vi "AlarmInterFace.vi"() -> ()   [LabVIEW 2015]
uses:
  <userlib>/QMH/Message Queue/Support/Enqueue Message (Single).vi
  <vilib>/Utility/error.llb/Error Cluster From Error Code.vi
  <vilib>/ErrorRing/Error Ring.xnode
  <userlib>/QMH/User Event - Stop/User Event - Stop.lvlib
  <userlib>/QMH/Message Queue/Message Queue.lvlib
panel:
  in  "报警声音消音":bool
  in  "确认所选报警":bool
  in  "确认当前画面所有报警":bool
  in  "AlarmMassge":i32(listbox)
  in  "Exit":bool
  in  "HostThread":variant
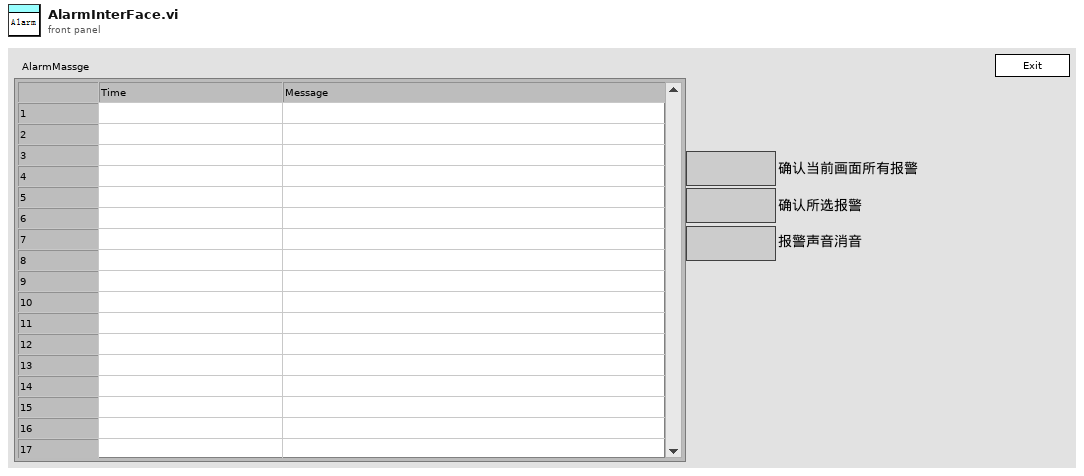
[diagram p1: front panel]
types:
  T1 = cluster{"Controls":cluster{"Exit":refnum<vi>, "AlarmMassge":refnum<vi>}, "Thread":cluster{"ThisQ":string, "ThisVI":refnum<vi>, "HostQ":string, "HostRef":refnum<vi>, "SlavesQ":string[], "SlavesRef":refnum<vi>[]}, "Data":cluster{"Replace":bool}, "User":cluster{"Name":string}}
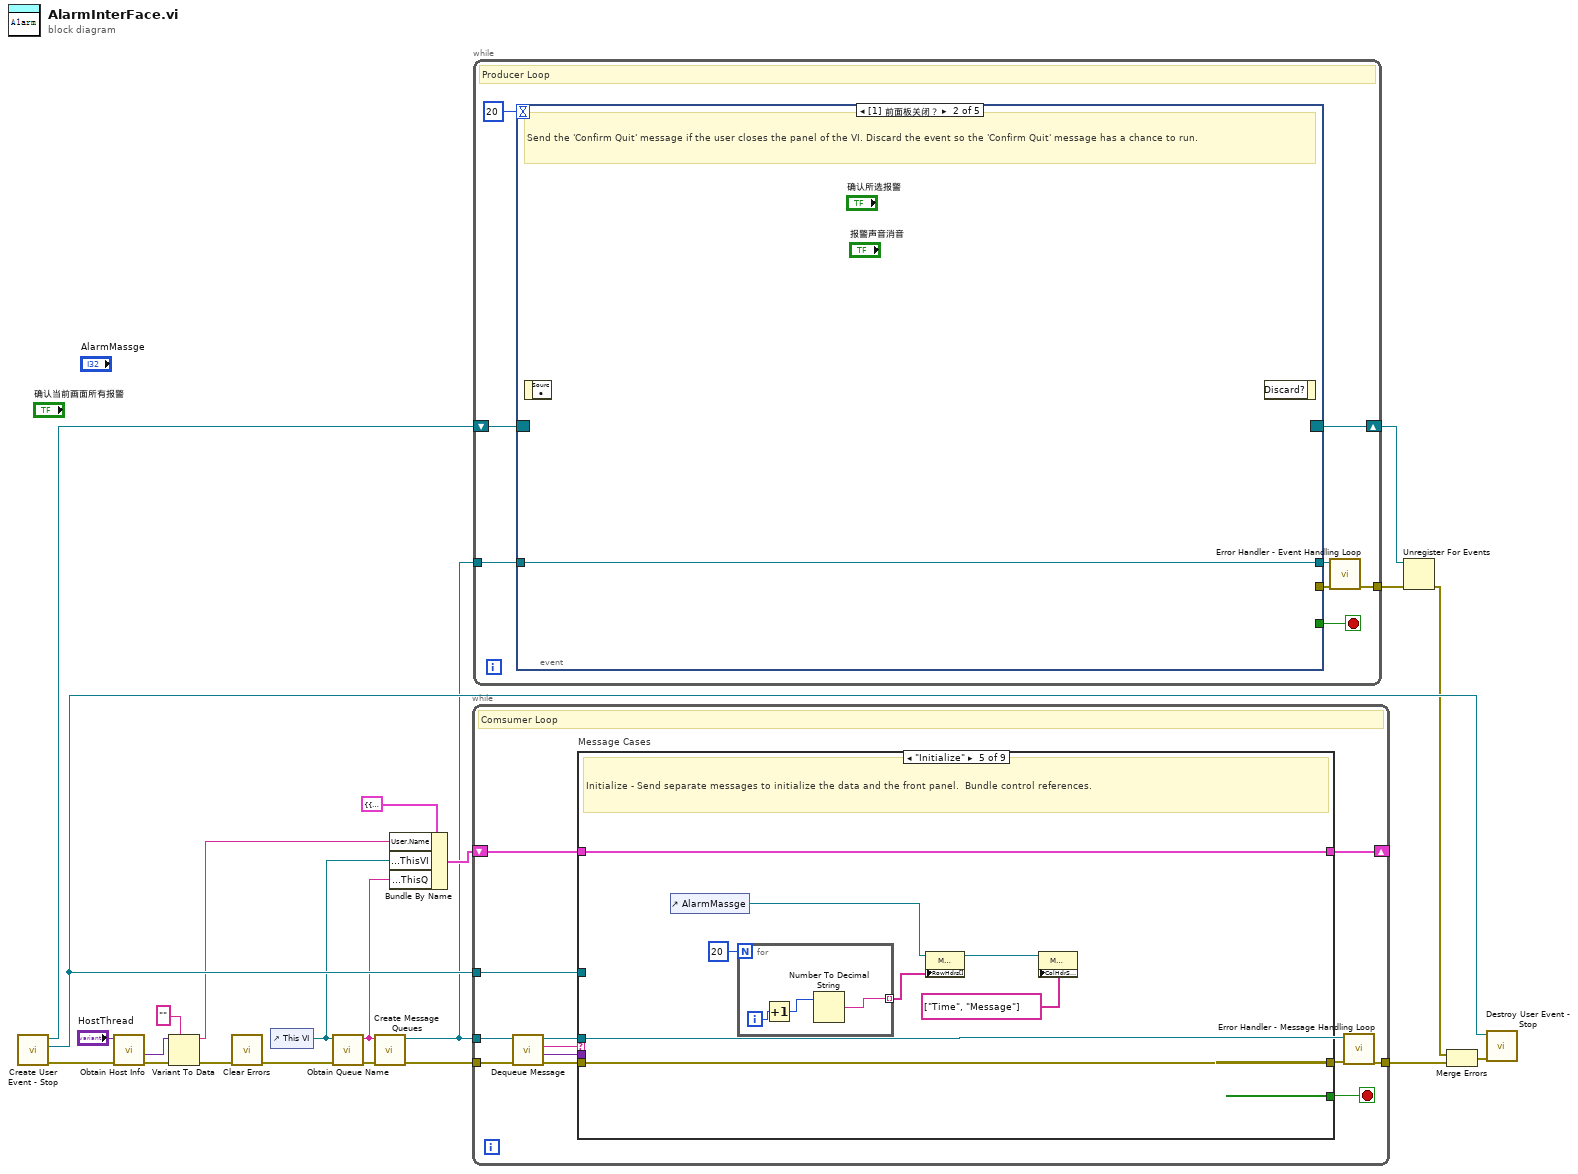
[diagram p0: block diagram]
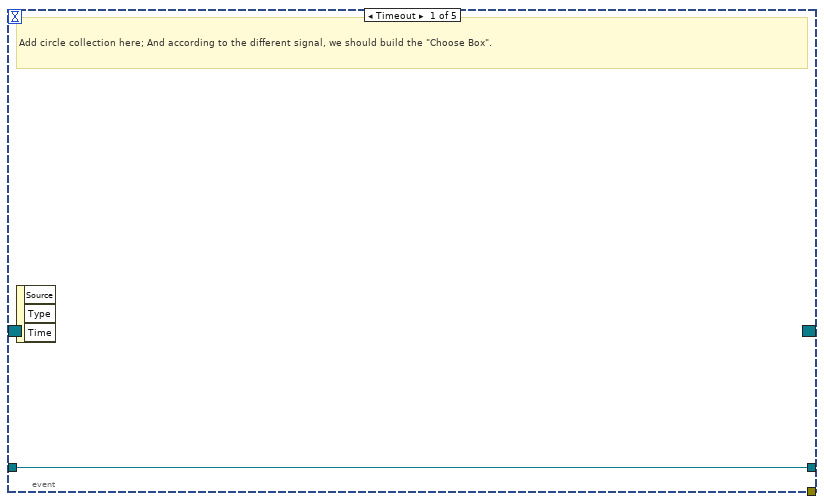
[diagram p2: hidden frame]
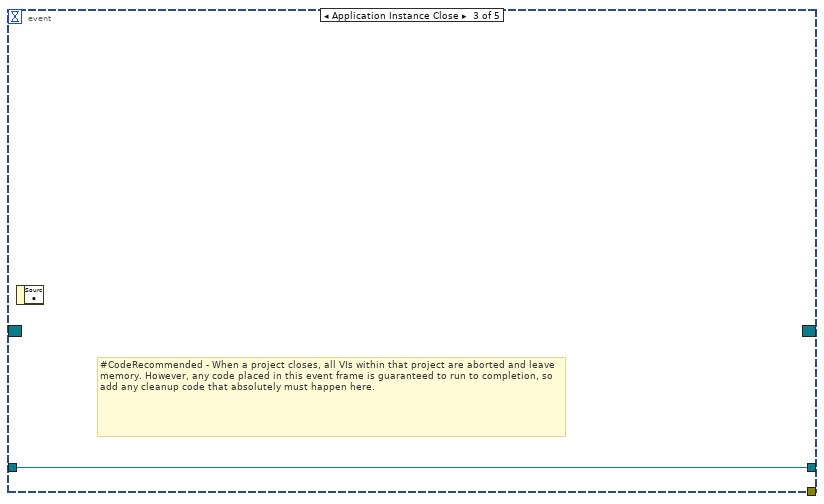
[diagram p3: hidden frame]
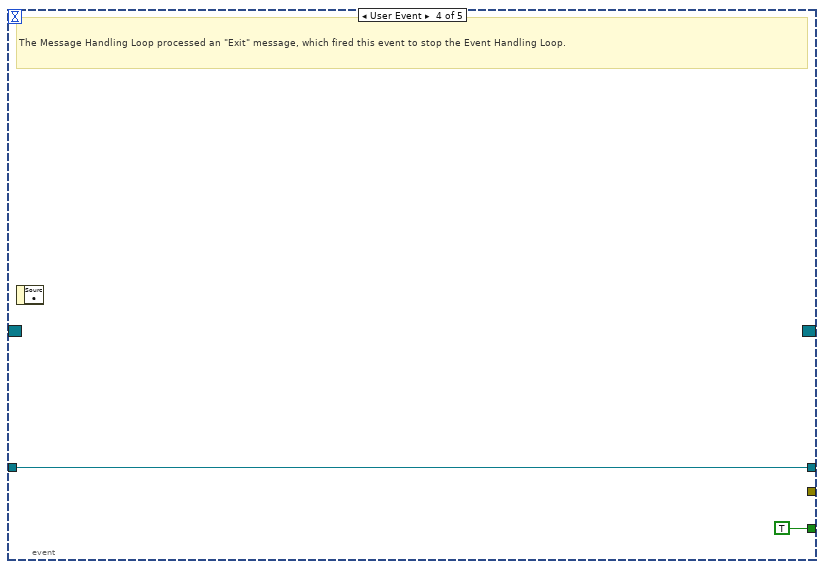
[diagram p4: hidden frame]
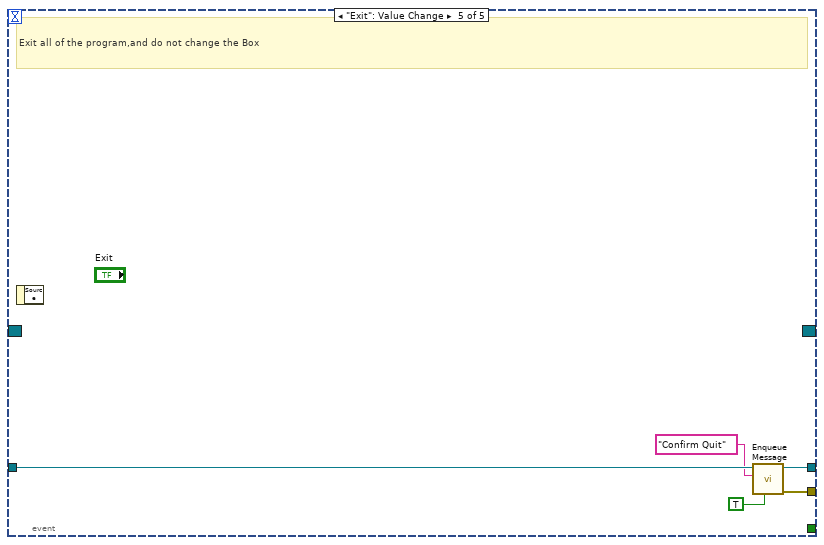
[diagram p5: hidden frame]
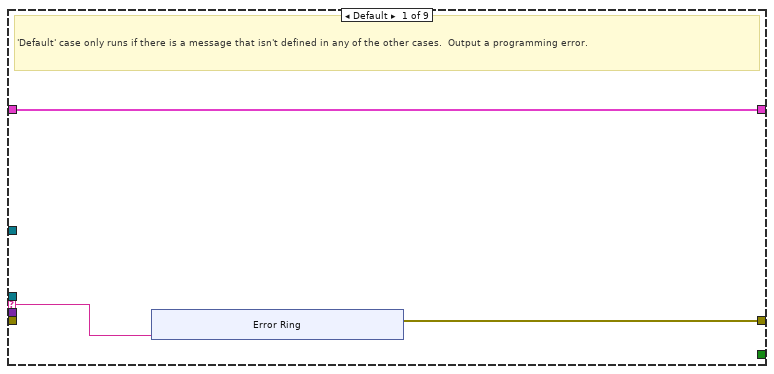
[diagram p6: hidden frame]
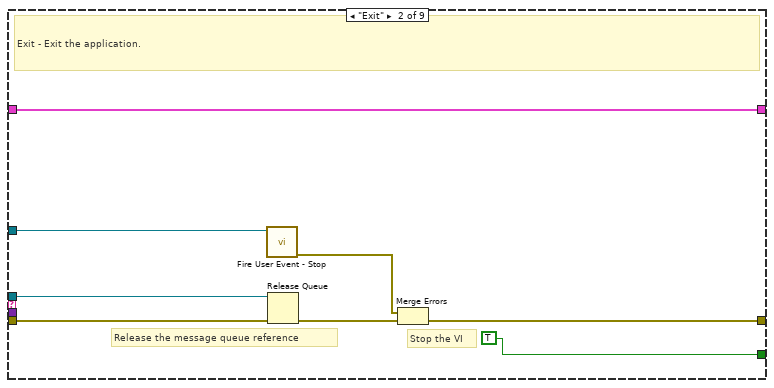
[diagram p7: hidden frame]
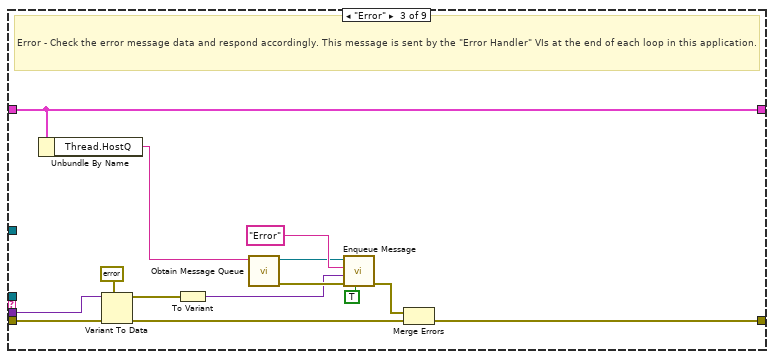
[diagram p8: hidden frame]
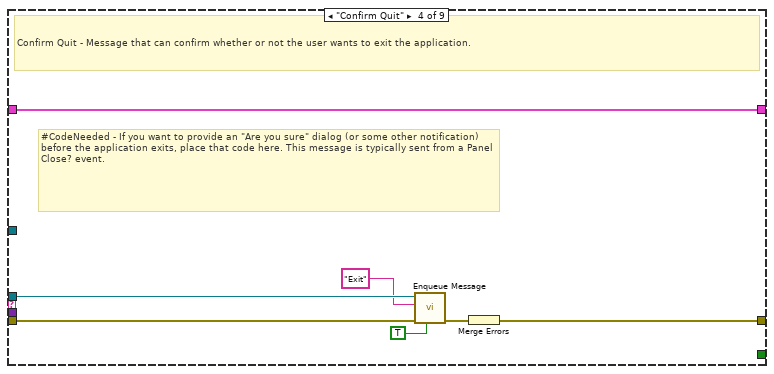
[diagram p9: hidden frame]
diagram:
  n1 = call <userlib>:"Create User Event - Stop.vi"() -> ("error out"=w9:errorcluster, "User Event - Stop"=w18:refnum<user-event>, "Stop Event Registration Refnum"=w20:refnum<event-registration>)  [unwired: 9 in]
  n2 = call <userlib>:"Obtain Host Info.vi"("error in (no error)"=w9, "HostThread"="HostThread") -> ("error out"=w6:errorcluster, "Data"=w5:variant)  [unwired: 6 in, 2 out]
  n3 = Variant To Data(error in=w6, type="", Variant=w5) -> (data=w1:string, error out=w3:errorcluster)
  n4 = call <vilib>:"Clear Errors.vi"("error in (no error)"=w3) -> ("error out"=w2:errorcluster)  [unwired: 5 in, 1 out]
  n5 = control-ref of="This VI"() -> (w11:refnum<vi>)
  n6 = call <userlib>:"Obtain Queue Name.vi"("error in (no error)"=w2, "VI Refnum"=w11) -> ("error out"=w14:errorcluster, "ViName"=w10:string)  [unwired: 8 in]
  n7 = call <userlib>:"Create Message Queues.vi"("error in (no error)"=w14, "name (unnamed)"=w10) -> ("error out"=w22:errorcluster, "QueueHandler"=w7:refnum<queue>)  [unwired: 8 in]
  n8 = Bundle By Name(cluster=T1 {"Controls"={"Exit"=refnum, "AlarmMassge"=refnum}, "Thread"={"ThisQ"="", "ThisVI"=refnum, "HostQ"="", "HostRef"=refnum, "SlavesQ"=[], "SlavesRef"=[]}, "Data"={"Replace"=FALSE}, "User"={"Name"=""}} ("Data Cluster"), "User.Name"=w1, "Thread.ThisVI"=w11, "Thread.ThisQ"=w10) -> (w12:T1)
  n9 = while {
    tunnel: w7 -> [w26]
    shift-right: [w33] -> _
    shift-left: w12 -> [w34]
    tunnel: w18 -> [w31]
    tunnel: w22 -> [w30]
    tunnel: [w24] -> w21
    stop <- w32 stop-if-true
    # "Comsumer Loop"
    n10 = call <userlib>:"Dequeue Message.vi"("error in (no error)"=w30, "Message Queue"=w26) -> ("error out"=w29:errorcluster, "Message Data"=w27:variant, "Message"=w28:string, "dup Message Queue"=w25:refnum<queue>)  [unwired: 6 in]
    n11 = case "Message Cases" shown="\"Initialize\"" w28 {
      selector: w28 -> [w35 _ _ _ _ _ _ _ _]
      tunnel: w25 -> [_ w52 _ w69 _ _ _ _ _]
      tunnel: w29 -> [_ w48 w66 w73 w79 w85 w87 w88 w91]
      tunnel: [w36 w49 w61 w71 w79 w85 w87 w88 w91] -> w23
      tunnel: w34 -> [w37 w45 w58 w72 w80 w84 w86 w89 w90]
      tunnel: [w37 w45 w58 w72 w80 w84 w86 w89 w90] -> w33
      tunnel: [_ TRUE _ _ _ _ _ _ _] -> w32
      tunnel: w27 -> [_ _ w65 _ _ _ _ _ _]
      tunnel: w31 -> [_ w47 _ _ _ _ _ _ _]
      frame Default {
        # "'Default' case only runs if there is a message that isn't defined in any of the other cases.  Output a programming error."
        n12 = xnode "Error Ring"("参数 0"=w35) -> ("错误输出"=w36:errorcluster)
      }
      frame "Exit" {
        # "Stop the VI"
        # "Release the message queue reference"
        # "Exit - Exit the application."
        n13 = call <userlib>:"Fire User Event - Stop.vi"("User Event - Stop"=w47) -> ("error out"=w46:errorcluster)  [unwired: 10 in]
        n14 = Release Queue(queue=w52, error in (no error)=w48) -> (error out=w50:errorcluster)  [unwired: 1 in, 2 out]
        n15 = Merge Errors(w46, w50) -> (w49:errorcluster)
      }
      frame "Error" {
        # "Error - Check the error message data and respond accordingly. This message is sent by the \"Error Handler\" VIs at the end of each loop in this application."
        n16 = Unbundle By Name(w58) -> ("Thread.HostQ"=w57:string)
        n17 = Variant To Data(error in=w66, type=errorcluster {"status"=FALSE, "code"=0, "source"=""} ("error constant"), Variant=w65) -> (data=w54:errorcluster, error out=w63:errorcluster)
        n18 = To Variant(anything=w54) -> (Variant=w53:variant)
        n19 = call <userlib>:"Obtain Message Queue.vi"("name (unnamed)"=w57) -> ("error out"=w56:errorcluster, "Message Queue"=w55:refnum<queue>)  [unwired: 9 in]
        n20 = call-poly <userlib>:"Enqueue Message.vi"("Priority Message? (F)"=TRUE, "error in (no error)"=w56, "Message Data"=w53, "Message"="Error", "Message Queue"=w55) -> ("error out"=w62:errorcluster)  [unwired: 5 in, 1 out]
        n21 = Merge Errors(w62, w63) -> (w61:errorcluster)
      }
      frame "Confirm Quit" {
        # "#CodeNeeded - If you want to provide an \"Are you sure\" dialog (or some other notification) before the application exits, place that code here. This message is typically sent from a Panel Close? event."
        # "Confirm Quit - Message that can confirm whether or not the user wants to exit the application."
        n22 = call-poly <userlib>:"Enqueue Message.vi"("Priority Message? (F)"=TRUE, "error in (no error)"=w73, "Message"="Exit", "Message Queue"=w69) -> ("error out"=w70:errorcluster)  [unwired: 6 in, 1 out]
        n23 = Merge Errors(w70) -> (w71:errorcluster)
      }
      frame "Initialize" {
        # "Initialize - Send separate messages to initialize the data and the front panel.  Bundle control references."
        n24 = control-ref of="AlarmMassge"() -> (w78:refnum<vi>)
        n25 = for {
          N: 20 -> [_]
          tunnel: [w83] -> w77 mode=indexing
          i -> [w82]
          n26 = Increment(x=w82) -> (x+1=w81:i32)
          n27 = Number To Decimal String(number=w81) -> (decimal integer string=w83:string)  [unwired: 1 in]
        }
        n28 = property class="MCListbox (严格)"(reference=w78, "RowHdrs[]"=w77) -> (reference out=w75:refnum<vi>)  [unwired: 1 in, 1 out]
        n29 = property class="MCListbox (严格)"(reference=w75, "ColHdrString"=string[] ["Time", "Message"]) -> ()  [unwired: 1 in, 2 out]
      }
      frame "<-------UI-------->" {
      }
      frame "<------Core------>" {
      }
      frame "Core_InitializeRef" {
        # "Initialize control references. For there is not enough space to locate all the control references, separate the codes into 2 messages"
      }
      frame "<---Operation--->" {
      }
    }
    n30 = call <userlib>:"Error Handler - Message Handling Loop.vi"("error in (no error)"=w23, "Message Queue"=w25) -> ("dup error in"=w24:errorcluster)  [unwired: 8 in, 1 out]
  }
  n31 = while {
    tunnel: w7 -> [w99]
    shift-right: [w97] -> w16
    shift-left: w20 -> [w98]
    tunnel: [w93] -> w15
    stop <- w95 stop-if-true
    # "Producer Loop"
    n32 = event shown="[1] 前面板关闭？" {
      selector: w98 -> [_ _ _ _ _]
      dyn-events: [_ _ _ _ _] -> w97
      timeout: 20 -> [_ _ _ _ _]
      tunnel: [_ _ _ TRUE ("Discard?") _] -> w95
      tunnel: w99 -> [w100 w101 w102 w104 w109]
      tunnel: [_ _ _ _ w107] -> w96
      tunnel: [w100 w101 w102 w104 w108] -> w94
      event Timeout {
        # "Add circle collection here; And according to the different signal, we should build the \"Choose Box\"."
        n33 = event-data() -> ()  [unwired: 1 in, 3 out]
      }
      event Panel Close? {
        # "Send the 'Confirm Quit' message if the user closes the panel of the VI. Discard the event so the 'Confirm Quit' message has a chance to run."
        n34 = event-data() -> ()  [unwired: 1 in, 1 out]
        n35 = event-data() -> ()  [unwired: 2 in, 1 out]
      }
      event Application Instance Close {
        # "#CodeRecommended - When a project closes, all VIs within that project are aborted and leave memory. However, any code placed in this event frame is guaranteed to run to completion, so add any cleanup code that absolutely must happen here."
        n36 = event-data() -> ()  [unwired: 1 in, 1 out]
      }
      event User Event {
        # "The Message Handling Loop processed an \"Exit\" message, which fired this event to stop the Event Handling Loop."
        n37 = event-data() -> ()  [unwired: 1 in, 1 out]
      }
      event "Exit": Value Change {
        # "Exit all of the program,and do not change the Box"
        n38 = event-data() -> ()  [unwired: 1 in, 1 out]
        n39 = call-poly <userlib>:"Enqueue Message.vi"("Priority Message? (F)"=TRUE, "Message"="Confirm Quit", "Message Queue"=w109) -> ("error out"=w107:errorcluster, "dup Message Queue"=w108:refnum<queue>)  [unwired: 7 in]
      }
    }
    n40 = call <userlib>:"Error Handler - Event Handling Loop.vi"("error in (no error)"=w96, "Message Queue"=w94) -> ("dup error in"=w93:errorcluster)  [unwired: 8 in, 1 out]
  }
  n41 = Unregister For Events(event registration refnum=w16, error in=w15) -> (error out=w17:errorcluster)
  n42 = Merge Errors(w17, w21) -> (w19:errorcluster)
  n43 = call <userlib>:"Destroy User Event - Stop.vi"("error in (no error)"=w19, "User Event - Stop"=w18) -> ()  [unwired: 9 in, 1 out]
